vi "Grabber Angles to Position.vi"() -> ()   [LabVIEW 2017]
panel:
  out "Y Final":dbl
  out "X Final":dbl
  in  "Lower Arm Angle Degrees":dbl
  in  "Upper Arm Angle Degrees":dbl
  in  "Lower Arm Length":dbl
  in  "Upper Arm Length":dbl
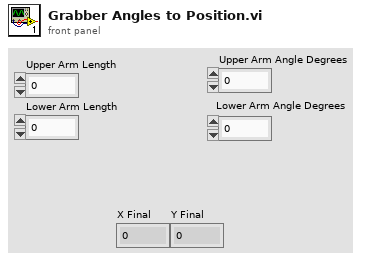
[diagram p1: front panel]
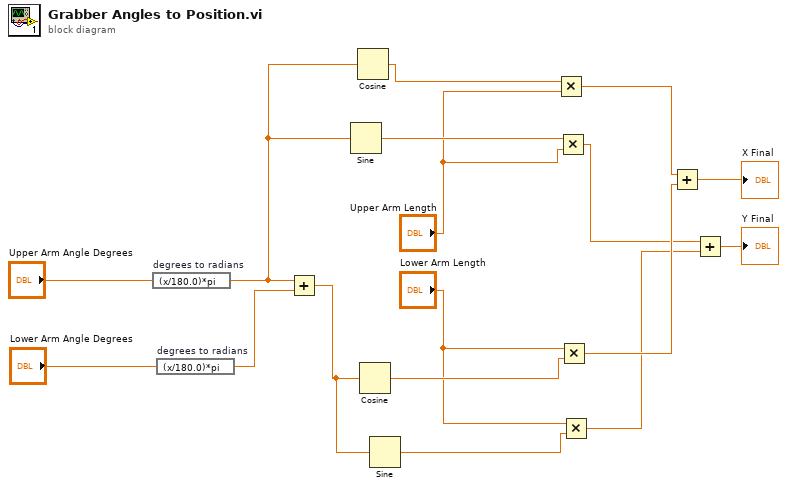
[diagram p0: block diagram]
diagram:
  n1 = expression code="(x/180.0)*pi" "degrees to radians"("Upper Arm Angle Degrees") -> (w15:dbl)
  n2 = expression code="(x/180.0)*pi" "degrees to radians"("Lower Arm Angle Degrees") -> (w13:dbl)
  n3 = Add(x=w15, y=w13) -> (x+y=w17:dbl)
  n4 = Sine(x=w15) -> (sin(x)=w11:dbl)
  n5 = Cosine(x=w15) -> (cos(x)=w16:dbl)
  n6 = Cosine(x=w17) -> (cos(x)=w9:dbl)
  n7 = Sine(x=w17) -> (sin(x)=w7:dbl)
  n8 = Multiply(x=w16, y="Upper Arm Length") -> (x*y=w6:dbl)
  n9 = Multiply(x=w11, y="Upper Arm Length") -> (x*y=w3:dbl)
  n10 = Multiply(x="Lower Arm Length", y=w9) -> (x*y=w5:dbl)
  n11 = Multiply(x="Lower Arm Length", y=w7) -> (x*y=w1:dbl)
  n12 = Add(x=w6, y=w5) -> (x+y=→"X Final":dbl)
  n13 = Add(x=w3, y=w1) -> (x+y=→"Y Final":dbl)
